vi "ConfigureDlg.vi"(8 "error in (no error)":errorcluster, 11 "C37.118 PMU in":refnum<class "C37.118 PMU.lvclass">) -> (0 "error out":errorcluster, 2 "Changed":bool, 3 "C37.118 PMU out":refnum<class "C37.118 PMU.lvclass">)   [LabVIEW 2014, in "SensorPlugins.lvlib" / "C37.118 PMU.lvclass"]
uses:
  C37.118 PMU.lvclass
  Typedef/PMUComms.ctl
  Typedef/eCommsType.ctl
  PmuBaseClass/Typedef/PmuConfig.ctl
  PmuBaseClass/Typedef/ePhases.ctl
  PmuBaseClass/PmuBase.lvclass/PmuBase.ctl
  C37.118 PMU.lvclass/C37.118 PMU.ctl
  <userlib>/NIST/BaseClasses/BasePlugin_class/BasePlugin.lvclass/BasePlugin.ctl
  PmuBaseClass/Accessors/Write PmuConfig.vi
  PmuBaseClass/Accessors/Write PhaseArray.vi
  Accessors/Write PMUComms.vi
  <userlib>/NIST/BaseClasses/BasePlugin_class/Accessors/Read PluginIniFilePath.vi
  PmuBaseClass/Accessors/Read PmuConfig.vi
  Accessors/Read PMUConfigData.vi
  PmuBaseClass/Accessors/Read PhaseArray.vi
  Accessors/Read PMUComms.vi
  <vilib>/Utility/config.llb/NI_LVConfig.lvlib
  <userlib>/NIST/NISTErrorLib/NISTErrorLib.lvlib
  PmuBaseClass/PmuBase.lvclass
panel:
  in  "btnGetConfig":bool
  in  "BtnDone":bool
  in  "PhaseArray":T1[](array[typedef])=[enum."VA", enum."VB", enum."VC", enum."V+", enum."IA", enum."IB", enum."IC", enum."I+"]
  in  "PmuConfig":T2={"Class"=enum."M", "Fs"=60, "F0"=60, "FSamp"=60, "SettlingTime"=0.0, "T0"=0.0}
  in  "PMUComms":T3={"PMU IP Address"="192.92.92.92", "CMD Comms Type"=enum."TCP", "Data Comms Type"=enum."TCP", "CMD Port"=4712, "Data Port"=4712, "PMU ID"=1}
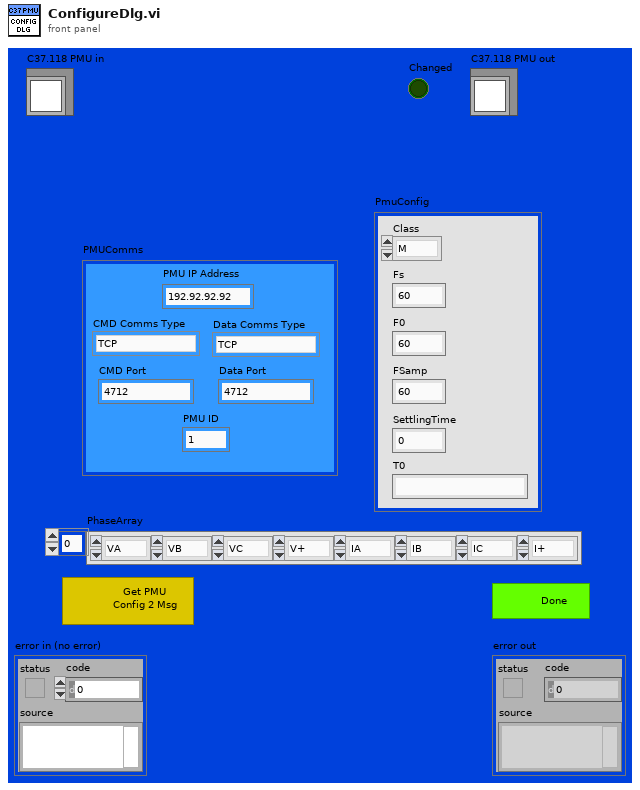
[diagram p1: front panel]
types:
  T1 = typedef "SensorPlugins.lvlib/PmuBase.lvclass/ePhases.ctl" = enum16{"VA", "VB", "VC", "V+", "IA", "IB", "IC", "I+", "none"}
  T2 = typedef "SensorPlugins.lvlib/PmuBase.lvclass/PmuConfig.ctl" = cluster{"Class":enum16{"M", "P"}, "Fs":i32, "F0":i32, "FSamp":i32, "SettlingTime":dbl, "T0":ext}
  T3 = typedef "SensorPlugins.lvlib/C37.118 PMU.lvclass/PMUComms.ctl" = cluster{"PMU IP Address":string, "CMD Comms Type":T4, "Data Comms Type":T4, "CMD Port":u16, "Data Port":u16, "PMU ID":u16}
  T4 = typedef "SensorPlugins.lvlib/C37.118 PMU.lvclass/eCommsType.ctl" = enum16{"TCP", "UDP", "USB", "GPIB"}
  T5 = enum32{"Invalid", "Standard", "Closed", "Hidden", "Minimized", "Maximized"}
  T6 = enum32{"Invalid", "Default", "Floating", "Floating/Auto-Hide", "Modal"}
  T7 = typedef "NI_LVConfig.lvlib/Config Data RefNum.ctl" = refnum<k1>
  T8 = typedef "SensorPlugins.lvlib/C37.118 PMU.lvclass/PMUConfigData.ctl" = cluster{"TimeBase":u32, "NUM_PMU":u16, "Station Name":string, "IDCODE":u16, "PHRNMR":u16, "ANNMR":u16, "DIGNMR":u16, "FORMAT BITS":T9, "Valid Inputs":u16[], "DigitalStatusMask":u16[], "24bit_PHUNIT":i32[], "24bit_ANUNIT":u32[], "Analog Amplitude Setting":u32[], "Unit (Vor I)":u8[], "ChannelNames":string, "Fs":i16, "SOC ":u32, "FRACSEC":u32, "F0":sgl, "CFGCNT":u16}
  T9 = typedef "SensorPlugins.lvlib/C37.118 PMU.lvclass/FormatBits.ctl" = cluster{"Rect/Polar":bool, "Phasor Int/Float":bool, "Analog Int/Float":bool, "F/ROCOF Int/Float":bool}
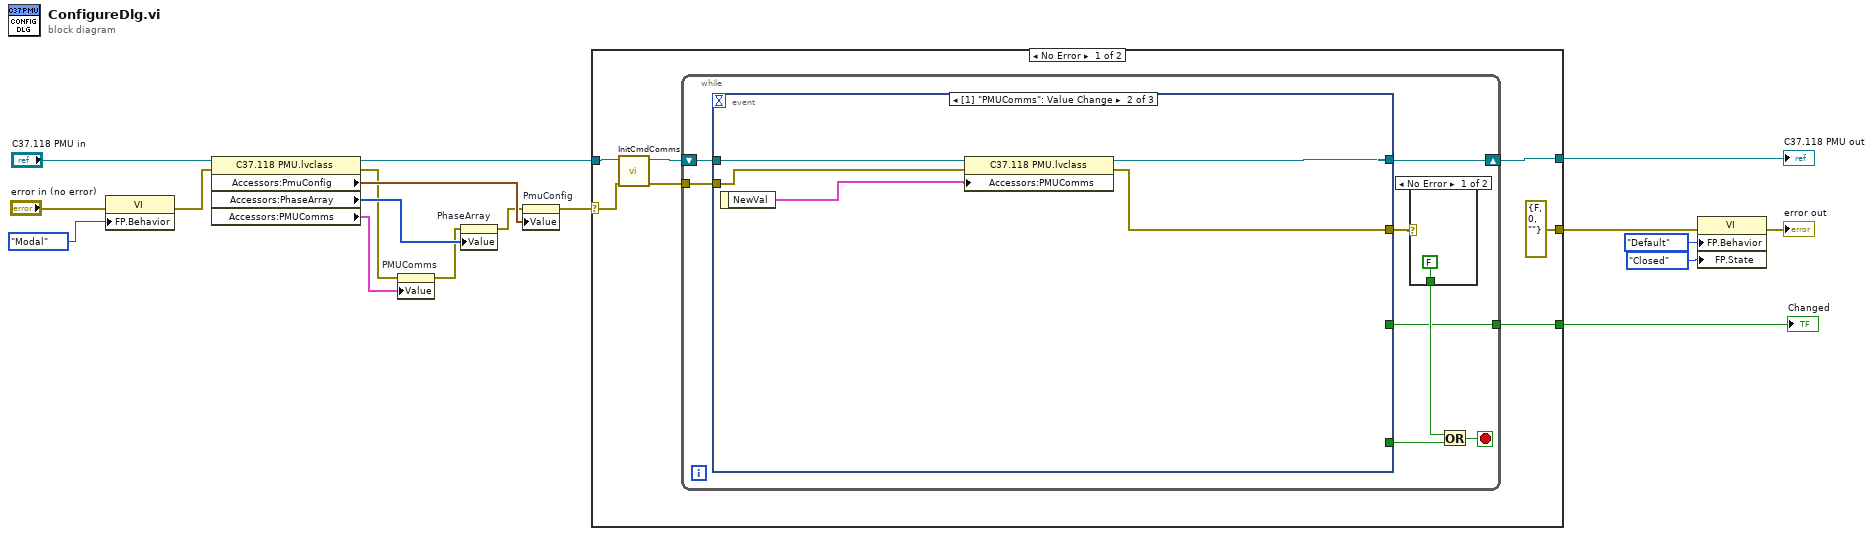
[diagram p0: block diagram]
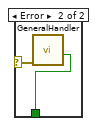
[diagram p2: hidden frame]
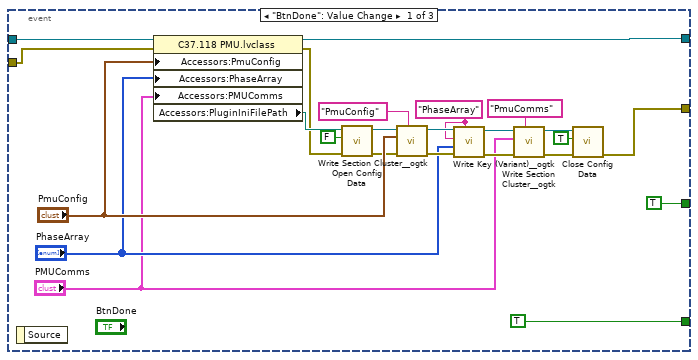
[diagram p3: hidden frame]
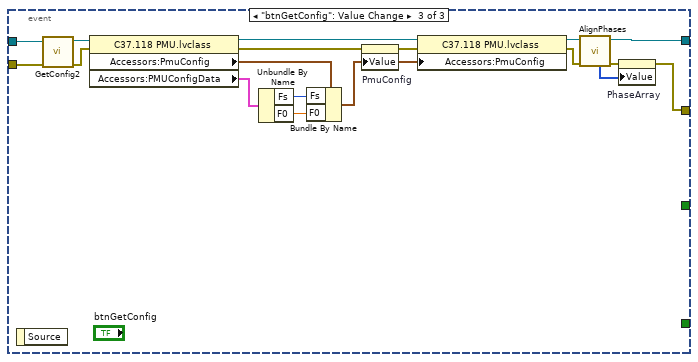
[diagram p4: hidden frame]
diagram:
  n1 = property class="VI"(error in="error in (no error)", "FP.Behavior"=T6."Modal" ("Front Panel Window:Behavior")) -> (error out=w5:errorcluster)  [unwired: 1 in, 1 out]
  n2 = property class="C37.118 PMU.lvclass"(reference="C37.118 PMU in", error in=w5) -> (reference out=w15:refnum<class "C37.118 PMU.lvclass">, error out=w11:errorcluster, "Accessors:PmuConfig"=w14:T2, "Accessors:PhaseArray"=w13:T1[], "Accessors:PMUComms"=w12:T3)
  n3 = property on="PMUComms" class="Clust (strict)"(error in=w11, "Value"=w12) -> (error out=w10:errorcluster)  [unwired: 1 in, 1 out]
  n4 = property on="PhaseArray" class="Arr (strict)"(error in=w10, "Value"=w13) -> (error out=w9:errorcluster)  [unwired: 1 in, 1 out]
  n5 = property on="PmuConfig" class="Clust (strict)"(error in=w9, "Value"=w14) -> (error out=w8:errorcluster)  [unwired: 1 in, 1 out]
  n6 = case shown="No Error" w8 {
    selector: w8 -> [w22 w84]
    tunnel: w15 -> [w24 w85]
    tunnel: [w25 w85] -> w17
    tunnel: [errorcluster {"status"=FALSE, "code"=0, "source"=""} ("error IO") w84] -> w16
    tunnel: [w19 _] -> w7
    frame No Error {
      n7 = call "InitCmdComms.vi"("error in (no error)"=w22, "C37.118 PMU in"=w24) -> ("error out"=w21:errorcluster, "C37.118 PMU out"=w23:refnum<class "C37.118 PMU.lvclass">)  [unwired: 8 in]
      n8 = while {
        shift-right: [w31] -> w25
        shift-left: w23 -> [w33]
        tunnel: w21 -> [w32]
        tunnel: [w26] -> w19
        stop <- w27 stop-if-true
        n9 = event shown="[1] \"PMUComms\": Value Change" {
          selector: _ -> [_ _ _]
          dyn-events: _ -> [_ _ _]
          timeout: _ -> [_ _ _]
          tunnel: w33 -> [w60 w65 w82]
          tunnel: w32 -> [w58 w64 w83]
          tunnel: [w39 w62 w68] -> w28
          tunnel: [TRUE _ _] -> w30
          tunnel: [w57 w61 w71] -> w31
          tunnel: [TRUE _ _] -> w26
          event "BtnDone": Value Change {
            w38 = "PhaseArray" ("section (optional)")
            n10 = event-data() -> ()  [unwired: 1 in, 1 out]
            n11 = property class="C37.118 PMU.lvclass"(reference=w60, error in=w58, "Accessors:PmuConfig"="PmuConfig", "Accessors:PhaseArray"="PhaseArray", "Accessors:PMUComms"="PMUComms") -> (reference out=w57:refnum<class "C37.118 PMU.lvclass">, error out=w54:errorcluster, "Accessors:PluginIniFilePath"=w56:path)
            n12 = call <vilib>:"Open Config Data.vi"("error in (no error)"=w54, "create file if necessary (T)"=FALSE, "configuration file path"=w56) -> ("error out"=w51:errorcluster, "refnum"=w53:T7)  [unwired: 6 in, 1 out]
            n13 = call <userlib>:"Write Section Cluster__ogtk.vi"("section (optional)"="PmuConfig", "error in (no error)"=w51, "Section Formatted Cluster"="PmuConfig", "refnum"=w53) -> ("error out"=w49:errorcluster, "dup refnum"=w48:T7)  [unwired: 6 in]
            n14 = call <userlib>:"Write Key (Variant)__ogtk.vi"("section"=w38, "error in (no error)"=w49, "key-value"="PhaseArray", "key (optional)"=w38, "refnum"=w48) -> ("error out"=w46:errorcluster, "refnum out"=w45:T7)  [unwired: 5 in]
            n15 = call <userlib>:"Write Section Cluster__ogtk.vi"("section (optional)"="PmuComms", "error in (no error)"=w46, "Section Formatted Cluster"="PMUComms", "refnum"=w45) -> ("error out"=w42:errorcluster, "dup refnum"=w41:T7)  [unwired: 6 in]
            n16 = call <vilib>:"Close Config Data.vi"("error in (no error)"=w42, "write file if changed (T)"=TRUE, "refnum"=w41) -> ("error out"=w39:errorcluster)  [unwired: 7 in, 1 out]
          }
          event Value Change {
            n17 = event-data() -> ("NewVal"=w63:T3)  [unwired: 1 in]
            n18 = property class="C37.118 PMU.lvclass"(reference=w65, error in=w64, "Accessors:PMUComms"=w63) -> (reference out=w61:refnum<class "C37.118 PMU.lvclass">, error out=w62:errorcluster)
          }
          event "btnGetConfig": Value Change {
            n19 = event-data() -> ()  [unwired: 1 in, 1 out]
            n20 = call "GetConfig2.vi"("error in (no error)"=w83, "C37.118 PMU in"=w82) -> ("error out"=w80:errorcluster, "C37.118 PMU out"=w81:refnum<class "C37.118 PMU.lvclass">)  [unwired: 8 in]
            n21 = property class="C37.118 PMU.lvclass"(reference=w81, error in=w80) -> (reference out=w78:refnum<class "C37.118 PMU.lvclass">, error out=w74:errorcluster, "Accessors:PmuConfig"=w77:T2, "Accessors:PMUConfigData"=w79:T8)
            n22 = Unbundle By Name(w79) -> ("Fs"=w76:i16, "F0"=w75:sgl)
            n23 = Bundle By Name(cluster=w77, "Fs"=w76, "F0"=w75) -> (w73:T2)
            n24 = property on="PmuConfig" class="Clust (strict)"(error in=w74, "Value"=w73) -> (error out=w66:errorcluster)  [unwired: 1 in, 1 out]
            n25 = property class="C37.118 PMU.lvclass"(reference=w78, error in=w66, "Accessors:PmuConfig"=w73) -> (reference out=w72:refnum<class "C37.118 PMU.lvclass">, error out=w70:errorcluster)
            n26 = call "AlignPhases.vi"("error in (no error)"=w70, "C37.118 PMU in"=w72) -> ("error out"=w69:errorcluster, "C37.118 PMU out"=w71:refnum<class "C37.118 PMU.lvclass">, "PhaseArray"=w67:T1[])  [unwired: 7 in]
            n27 = property on="PhaseArray" class="Arr (strict)"(error in=w69, "Value"=w67) -> (error out=w68:errorcluster)  [unwired: 1 in, 1 out]
          }
        }
        n28 = case shown="No Error" w28 {
          selector: w28 -> [_ w35]
          tunnel: [FALSE ("Stop") w36] -> w29
          frame No Error {
          }
          frame Error {
            n29 = call <userlib>:"GeneralHandler.vi"("error in (no error)"=w35) -> ("Stop"=w36:bool)  [unwired: 7 in, 3 out]
          }
        }
        n30 = Or(x=w29, y=w30) -> (x .or. y?=w27:bool)
      }
    }
    frame Error {
    }
  }
  "C37.118 PMU out" <- w17
  "Changed" <- w7
  n31 = property class="VI"(error in=w16, "FP.Behavior"=T6."Default" ("Front Panel Window:Behavior"), "FP.State"=T5."Closed" ("Front Panel Window:State")) -> (error out=→"error out":errorcluster)  [unwired: 1 in, 1 out]
